vi "Actor Core.vi"(8 "error in":errorcluster, 11 "Format Converter in":refnum<class "Format Converter.lvclass">) -> (0 "error out":errorcluster, 3 "Actor out":refnum<class "Actor.lvclass">)   [LabVIEW 2016, in "Format Converter.lvclass"]
doc: "(<B>Filename</B>: Actor Framework.lvlib:Actor.lvclass:Actor Core.vi)\n\nReceives messages to the actor, reacts to them, and initiates any error handling that may shut the actor down.\n\nDescendant classes may override this VI to append parallel tasks for the actor to complete while it handles messages. Overrides use the Call Parent Method node."
uses:
  Format Converter.lvclass
  C:/github/Measure_core/da Base/Template Module.lvclass
  C:/Program Files/National Instruments/LabVIEW 2016/vi.lib/ActorFramework/Actor/Actor.lvclass
  <vilib>/ActorFramework/Actor/Actor.lvclass
  NHMFL_Core/Libraries/File/File Format Converter/Format Converter Configuration.ctl
  Measure_core/Template Module/Template Module.lvclass/Template Module.ctl
  <vilib>/ActorFramework/Actor/Actor.lvclass/Actor.ctl
  <vilib>/ActorFramework/Message Enqueuer/Message Enqueuer.lvclass/Message Enqueuer.ctl
  Measure_core/Results/File Path Result/File Path Result.lvclass
  C:/github/Measure_core/Results/Acquired Result/Acquired Result.lvclass
  Measure_core/Process Object Messages/Process Result Msg/Process Result Msg.lvclass/Process Result Msg.ctl
  Measure_core/Template Module/Read stop event.vi
  <vilib>/ActorFramework/Message Enqueuer/Init from Existing Queue.vi
  <vilib>/ActorFramework/Message Enqueuer/Enqueue.vi
  Measure_core/Process Object Messages/Process Result Msg/Process Result Msg.lvclass
  C:/Program Files/National Instruments/LabVIEW 2016/vi.lib/ActorFramework/Message/Message.lvclass
  <vilib>/ActorFramework/Message Priority Queue/Priority Enqueue.vi
  Measure_core/Process Object/Process Object.lvclass
  <vilib>/ActorFramework/Message Enqueuer/Message Enqueuer.lvclass
panel:
  out "Output file":path
  in  "Input file":path
  in  "Re-process":bool
  out "Name":string
  in  "Configuration":T1={"New start time"=nan, "New end time"=nan, "Output file format"=enum."ASCII", "Save ASCII column names"=TRUE, "Prepend binary array size"=FALSE, "buffer size (-1: all)"=100000, "Channels"=[], "Group"="p", "New dt"=nan} {"buffer size (-1: all)" format="%.0p"; "New start time" format="%#_10p"}
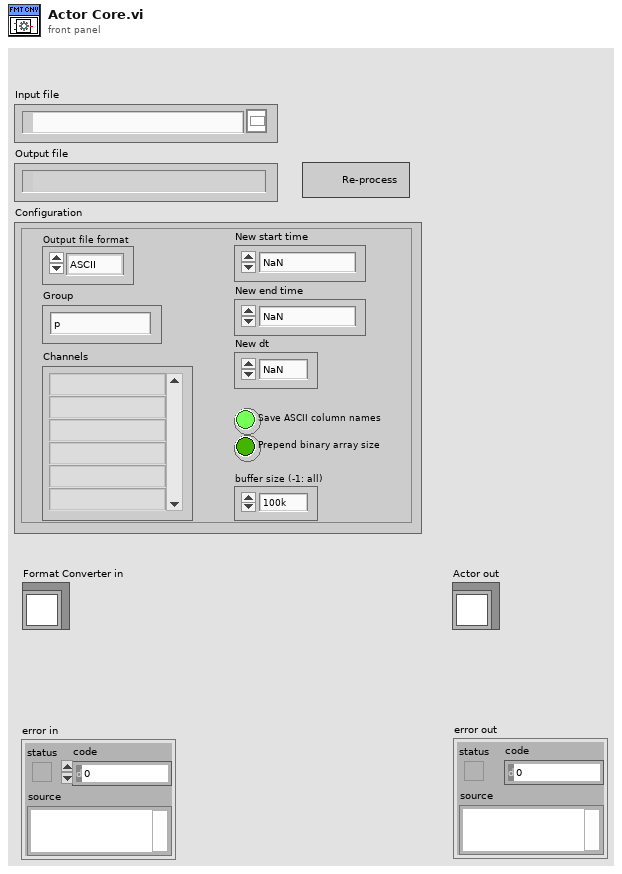
[diagram p1: front panel]
types:
  T1 = typedef "Format Converter Configuration.ctl" = cluster{"New start time":dbl, "New end time":dbl, "Output file format":enum16{"ASCII", "BINARY", "TDMS"}, "Save ASCII column names":bool, "Prepend binary array size":bool, "buffer size (-1: all)":i64, "Channels":string[], "Group":string, "New dt":dbl}
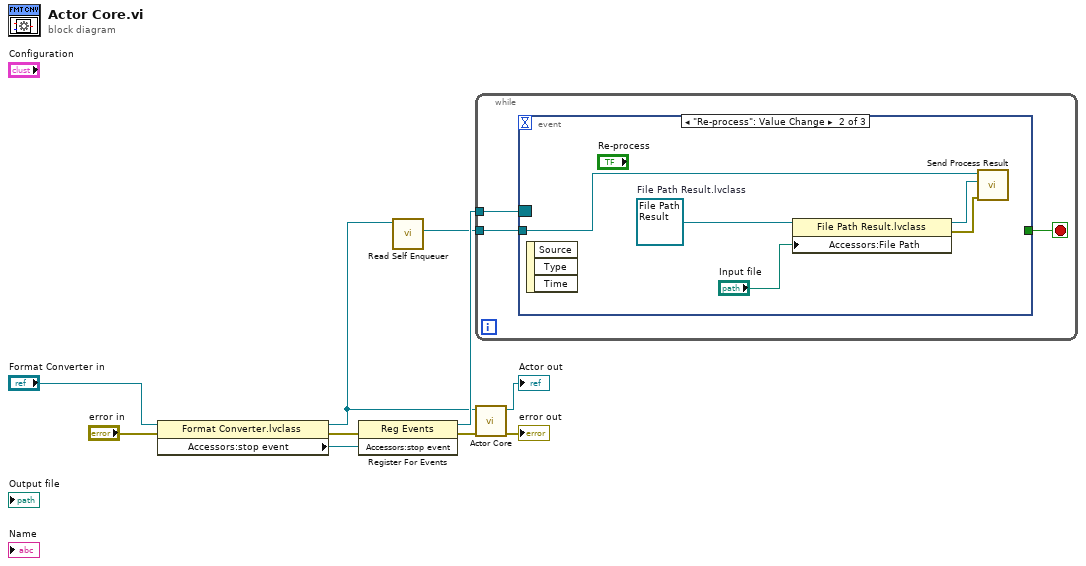
[diagram p0: block diagram]
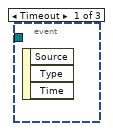
[diagram p2: hidden frame]
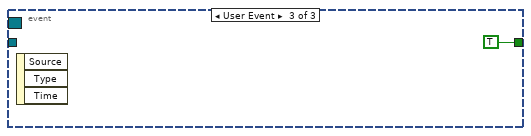
[diagram p3: hidden frame]
diagram:
  n1 = property class="Format Converter.lvclass"(reference="Format Converter in", error in="error in") -> (reference out=w1:refnum<class "Format Converter.lvclass">, error out=w8:errorcluster, "Accessors:stop event"=w7:refnum<user-event>)
  n2 = register-events(error in=w8, w7) -> (reference out=w3:refnum<event-registration>, error out=w4:errorcluster)  [unwired: 1 in]
  n3 = call <vilib>:"Read Self Enqueuer.vi"("Actor"=w1) -> ("Self Enqueuer"=w2:refnum<class "Message Enqueuer.lvclass">)  [unwired: 10 in]
  n4 = while {
    tunnel: w3 -> [w13]
    tunnel: w2 -> [w11]
    stop <- w12 stop-if-true
    n5 = event shown="[1] \"Re-process\": Value Change" {
      selector: w13 -> [_ _ _]
      dyn-events: _ -> [_ _ _]
      timeout: _ -> [_ _ _]
      tunnel: [_ _ TRUE] -> w12
      tunnel: w11 -> [_ w18 _]
      event Timeout {
        n6 = event-data() -> ()  [unwired: 1 in, 3 out]
      }
      event "Re-process": Value Change {
        w17 = refnum<class "File Path Result.lvclass"> refnum  # File Path Result.lvclass
        n7 = event-data() -> ()  [unwired: 1 in, 3 out]
        n8 = property class="File Path Result.lvclass"(reference=w17, "Accessors:File Path"="Input file") -> (reference out=w16:refnum<class "File Path Result.lvclass">, error out=w15:errorcluster)  [unwired: 1 in]
        n9 = call "Send Process Result.vi"("error in (no error)"=w15, "Result in"=w16, "Message Enqueuer"=w18) -> ()  [unwired: 7 in, 2 out]
      }
      event User Event {
        n10 = event-data() -> ()  [unwired: 1 in, 3 out]
      }
    }
  }
  n11 = call-parent "Actor Core.vi"("error in"=w4, "Measure Object in"=w1) -> ("error out"=→"error out":errorcluster, "Actor out"=→"Actor out":refnum<class "Actor.lvclass">)  [unwired: 8 in]
